vi "Laborator 5.vi"() -> ()   [LabVIEW 2023]
panel:
  out "?":bool
  in  "b":dbl
  in  "a":dbl
  out "Nr. valori negative":i32
  out "Nr. valori nule":i32
  out "Nr valori pozitive":i32
  out "Nr. valori intre a si b":i32
  in  "Array":dbl[](array[numeric])
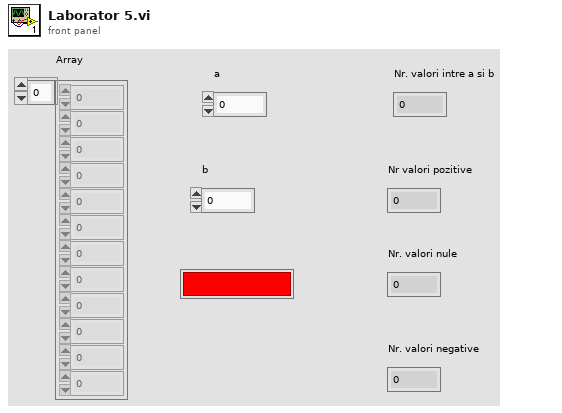
[diagram p1: front panel]
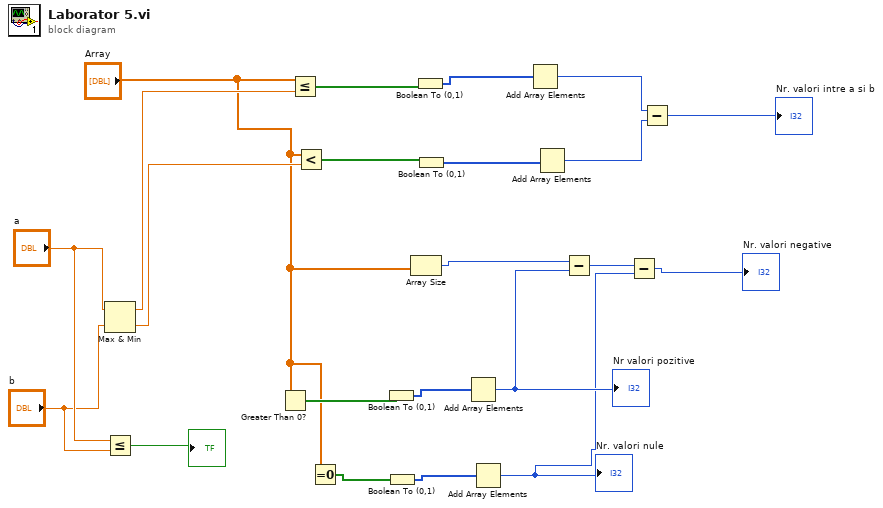
[diagram p0: block diagram]
diagram:
  n1 = Max & Min(x="a", y="b") -> (max(x,y)=w22:dbl, min(x,y)=w19:dbl)
  n2 = Less Or Equal?(x="a", y="b") -> (x <= y?=→"?":bool)
  n3 = Greater Than 0?(x="Array") -> (x > 0?=w13:bool[])
  n4 = Less Or Equal?(x="Array", y=w22) -> (x <= y?=w21:bool[])
  n5 = Less?(x="Array", y=w19) -> (x < y?=w18:bool[])
  n6 = Equal To 0?(x="Array") -> (x = 0?=w11:bool[])
  n7 = Boolean To (0,1)(Boolean=w13) -> (0, 1=w12:i16[])
  n8 = Boolean To (0,1)(Boolean=w11) -> (0, 1=w10:i16[])
  n9 = Array Size(array="Array") -> (size(s)=w8:i32)
  n10 = Boolean To (0,1)(Boolean=w21) -> (0, 1=w20:i16[])
  n11 = Boolean To (0,1)(Boolean=w18) -> (0, 1=w17:i16[])
  n12 = Add Array Elements(numeric array=w12) -> (sum=w7:i16)
  "Nr valori pozitive" <- w7
  n13 = Add Array Elements(numeric array=w10) -> (sum=w5:i16)
  "Nr. valori nule" <- w5
  n14 = Add Array Elements(numeric array=w20) -> (sum=w16:i16)
  n15 = Add Array Elements(numeric array=w17) -> (sum=w15:i16)
  n16 = Subtract(x=w8, y=w7) -> (x-y=w6:i32)
  n17 = Subtract(x=w6, y=w5) -> (x-y=→"Nr. valori negative":i32)
  n18 = Subtract(x=w16, y=w15) -> (x-y=→"Nr. valori intre a si b":i16)
